vi "DEPRECATED - 4ButtonsTo2 - David G.vi"(0 "False- 1":dbl, 1 "False 2":dbl, 2 "True-True 1":dbl, 3 "True-True 2":dbl, 4 "True-False-True 2":dbl, 5 "True-False-True 1":dbl, 6 "True-False-False 1":dbl, 7 "True-False-False 2":dbl, 11 "Button Pressed?":bool, 12 "Check Value 1":dbl, 14 "Check Value 2":dbl, 17 "Inverted?":bool, 20 "Encoder 1":string="My Encoder RefNum", 21 "Encoder 2":string="My Encoder RefNum", 22 "Motor 1":string="My Encoder RefNum", 23 "Motor 2":string="My Encoder RefNum") -> ()   [LabVIEW 2016]
panel:
  in  "Inverted?":bool
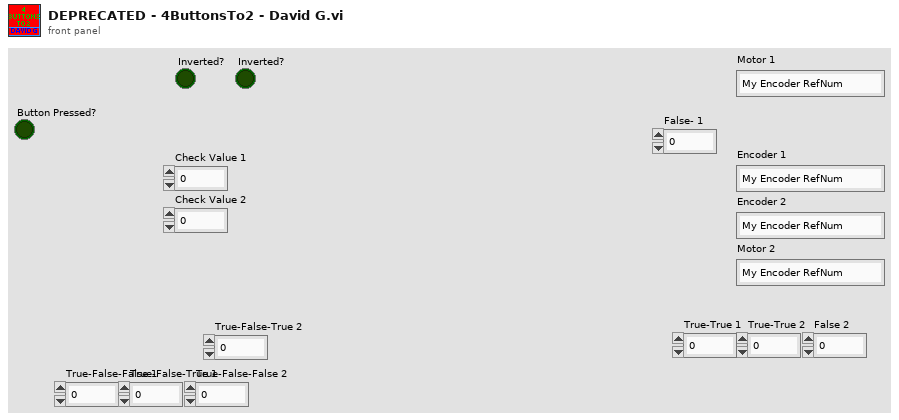
[diagram p1: front panel]
types:
  T1 = typedef "WPI_EncoderDevRef.ctl" = cluster{"DevStatus":errorcluster, "EncoderIndex":T2, "CounterIndex":T3, "DistancePerCount":dbl, "Decoding Type":T4}
  T2 = typedef "FPGA_EncoderIdx.ctl" = enum8{"Enc 0", "Enc 1", "Enc 2", "Enc 3", "Enc 4", "Enc 5", "Enc 6", "Enc 7", "Invalid"}
  T3 = typedef "FPGA_CounterCtrSystemIndex.ctl" = enum8{"Ctr 0", "Ctr 1", "Ctr 2", "Ctr 3", "Ctr 4", "Ctr 5", "Ctr 6", "Ctr 7", "Invalid"}
  T4 = typedef "WPI_EncoderType.ctl" = enum16{"1x", "2x", "4x"}
  T5 = typedef "WPI_MotorControlDeviceRef.ctl" = cluster{"DeviceStatus":errorcluster, "Type":T6, "PWM":cluster{"PWM Channel":T7, "DeadBand":T8}, "CAN":cluster{"Device Number":u8, "SetOutput VI Ref":variant, "GetOutput VI Ref":variant, "Enable VI Ref":variant, "Disable VI Ref":variant, "Data":variant}, "Invert":bool}
  T6 = typedef "WPI_MotorControlType.ctl" = enum16{"PWM", "CAN"}
  T7 = typedef "FPGA_DIOPWMChannel.ctl" = enum8{"PWM 0", "PWM 1", "PWM 2", "PWM 3", "PWM 4", "PWM 5", "PWM 6", "PWM 7", "PWM 8", "PWM 9", "PWM MXP 0", "PWM MXP 1", "PWM MXP 2", "PWM MXP 3", "PWM MXP 4", "PWM MXP 5", "PWM MXP 6", "PWM MXP 7", "PWM MXP 8", "PWM MXP 9", "Invalid"}
  T8 = typedef "WPI_PWMDeadband.ctl" = cluster{"Name":string, "maxPositivePwm":i32, "minPositivePwm":i32, "centerPwm":i32, "maxNegativePwm":i32, "minNegativePwm":i32, "angularRange":u16}
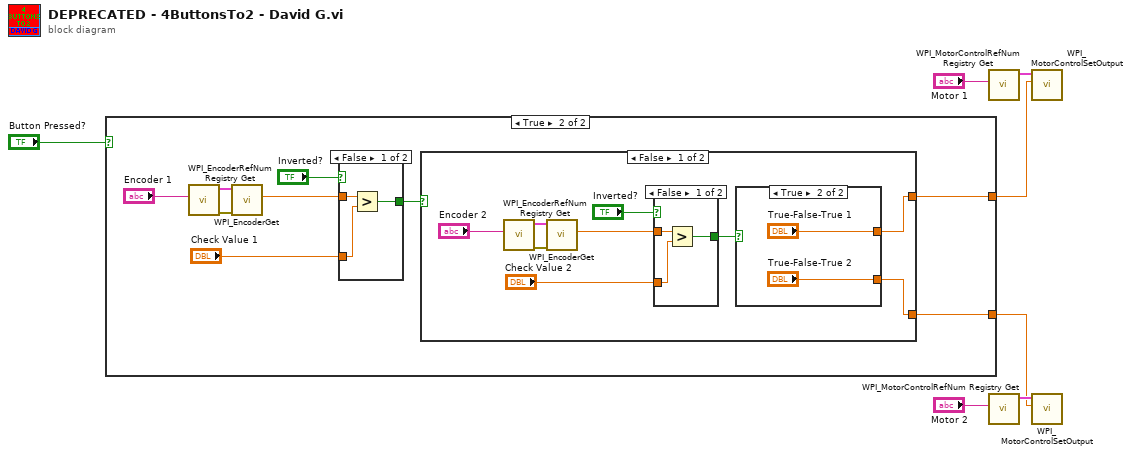
[diagram p0: block diagram]
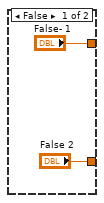
[diagram p2: hidden frame]
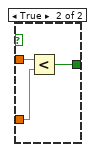
[diagram p3: hidden frame]
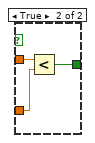
[diagram p4: hidden frame]
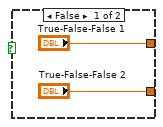
[diagram p5: hidden frame]
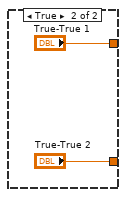
[diagram p6: hidden frame]
diagram:
  n1 = case shown="True" "Button Pressed?" {
    tunnel: ["False- 1" w14] -> w5
    tunnel: ["False 2" w13] -> w6
    frame False {
    }
    frame True {
      n2 = call <vilib>:"WPI_EncoderRefNum Registry Get.vi"("refnum name"="Encoder 1") -> ("error out"=w17:errorcluster, "EncoderDevRef"=w18:T1)  [unwired: 9 in]
      n3 = call <vilib>:"WPI_EncoderGet.vi"("error in (no error)"=w17, "EncoderDevRef"=w18) -> ("Distance"=w16:dbl)  [unwired: 4 in, 5 out]
      n4 = case shown="False" "Inverted?" {
        tunnel: w16 -> [w21 w24]
        tunnel: [w19 w23] -> w15
        tunnel: "Check Value 1" -> [w20 w22]
        frame False {
          n5 = Greater?(x=w21, y=w20) -> (0:w19:bool)
        }
        frame True {
          n6 = Less?(x=w24, y=w22) -> (x < y?=w23:bool)
        }
      }
      n7 = case shown="False" w15 {
        tunnel: [w28 "True-True 1"] -> w14
        tunnel: [w29 "True-True 2"] -> w13
        frame False {
          n8 = call <vilib>:"WPI_EncoderRefNum Registry Get.vi"("refnum name"="Encoder 2") -> ("error out"=w32:errorcluster, "EncoderDevRef"=w33:T1)  [unwired: 9 in]
          n9 = call <vilib>:"WPI_EncoderGet.vi"("error in (no error)"=w32, "EncoderDevRef"=w33) -> ("Distance"=w31:dbl)  [unwired: 4 in, 5 out]
          n10 = case shown="False" "Inverted?" {
            tunnel: w31 -> [w35 w39]
            tunnel: [w34 w38] -> w30
            tunnel: "Check Value 2" -> [w36 w37]
            frame False {
              n11 = Greater?(x=w35, y=w36) -> (0:w34:bool)
            }
            frame True {
              n12 = Less?(x=w39, y=w37) -> (x < y?=w38:bool)
            }
          }
          n13 = case shown="True" w30 {
            tunnel: ["True-False-False 2" "True-False-True 2"] -> w29
            tunnel: ["True-False-False 1" "True-False-True 1"] -> w28
            frame False {
            }
            frame True {
            }
          }
        }
        frame True {
        }
      }
    }
  }
  n14 = call <vilib>:"WPI_MotorControlRefNum Registry Get.vi"("refnum name"="Motor 1") -> ("MotorControlDevRef"=w3:T5)  [unwired: 9 in, 1 out]
  n15 = call <vilib>:"WPI_MotorControlRefNum Registry Get.vi"("refnum name"="Motor 2") -> ("MotorControlDevRef"=w7:T5)  [unwired: 9 in, 1 out]
  n16 = call <vilib>:"WPI_MotorControlSetOutput.vi"("Output"=w5, "MotorControlDevRef"=w3) -> ()  [unwired: 7 in, 3 out]
  n17 = call <vilib>:"WPI_MotorControlSetOutput.vi"("Output"=w6, "MotorControlDevRef"=w7) -> ()  [unwired: 7 in, 3 out]
